vi "Detect window length change.vi"(11 "NewRange":T1) -> (3 "Window length changed":bool)   [LabVIEW 2013, in "XGrapher.xctl"]
uses:
  XGrapher.xctl
  <vilib>/Utility/miscctls.llb/LVRangeTypeDef.ctl
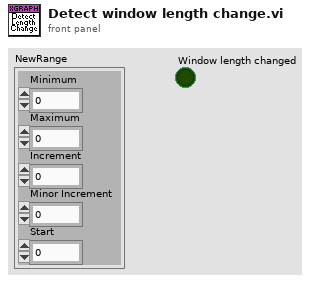
[diagram p1: front panel]
types:
  T1 = typedef "LVRangeTypeDef.ctl" = cluster{"Minimum":dbl, "Maximum":dbl, "Increment":dbl, "Minor Increment":dbl, "Start":dbl}
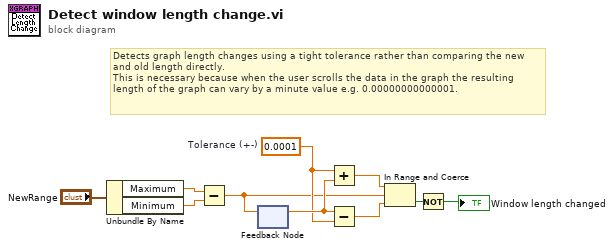
[diagram p0: block diagram]
diagram:
  w2 = 0.0001  # Tolerance (+-)
  # "Detects graph length changes using a tight tolerance rather than comparing the new and old length directly.\nThis is necessary because when the user scrolls the data in the graph the resulting length of the graph can vary by a minute value e.g. 0.00000000000001."
  n1 = Unbundle By Name("NewRange") -> ("Maximum"=w4:dbl, "Minimum"=w5:dbl)
  n2 = Subtract(x=w4, y=w5) -> (x-y=w1:dbl)
  n3 = feedback #1() -> (w3:dbl)  [unwired: 1 in]
  n4 = feedback-in #1(w1) -> ()
  n5 = Add(x=w2, y=w3) -> (x+y=w7:dbl)
  n6 = Subtract(x=w3, y=w2) -> (x-y=w8:dbl)
  n7 = In Range and Coerce(upper limit=w7, x=w1, lower limit=w8) -> (In Range?=w9:bool)  [unwired: 1 out]
  n8 = Not(x=w9) -> (.not. x?=→"Window length changed":bool)
